vi "main.vi"() -> ()   [LabVIEW 2018]
uses:
  global.vi
  <vilib>/Instr/_visa.llb/VISA Configure Serial Port (Instr).vi
panel:
  out "当前位置":dbl
  out "频率test":string
  out "开关test":string
  out "步进电机test":string
  in  "停止":bool
  in  "改变开关":dbl=1.0 min=1.0 max=31.0 step=1.0
  in  "连接开关控制器":refnum<visa-resource-name>
  in  "连接步进电机控制器":refnum<visa-resource-name>
  in  "改变频率":dbl=24.0
  in  "改变位置":dbl
  in  "暂停":bool
  in  "开始":bool
  out "当前开关":dbl
  out "当前频率":dbl
  in  "扫描模式":string(combo)="多频多角度扫描"
  in  "测量距离/mm":dbl=150.0
  in  "频率步进/GHz":dbl=0.1
  in  "截止频率/GHz":dbl=30.0
  in  "起始频率/GHz":dbl=24.0
  in  "电机步进/mm":dbl=5.0
  in  "电机长度/mm":dbl=200.0
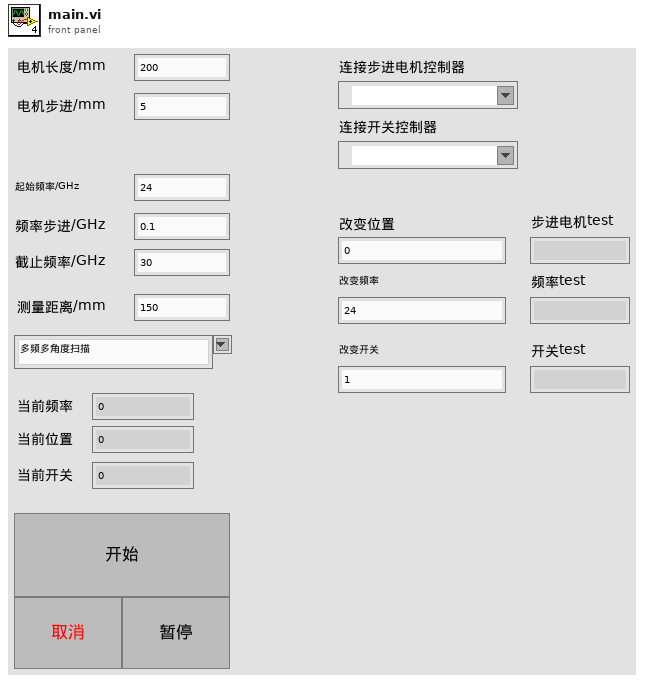
[diagram p1: front panel]
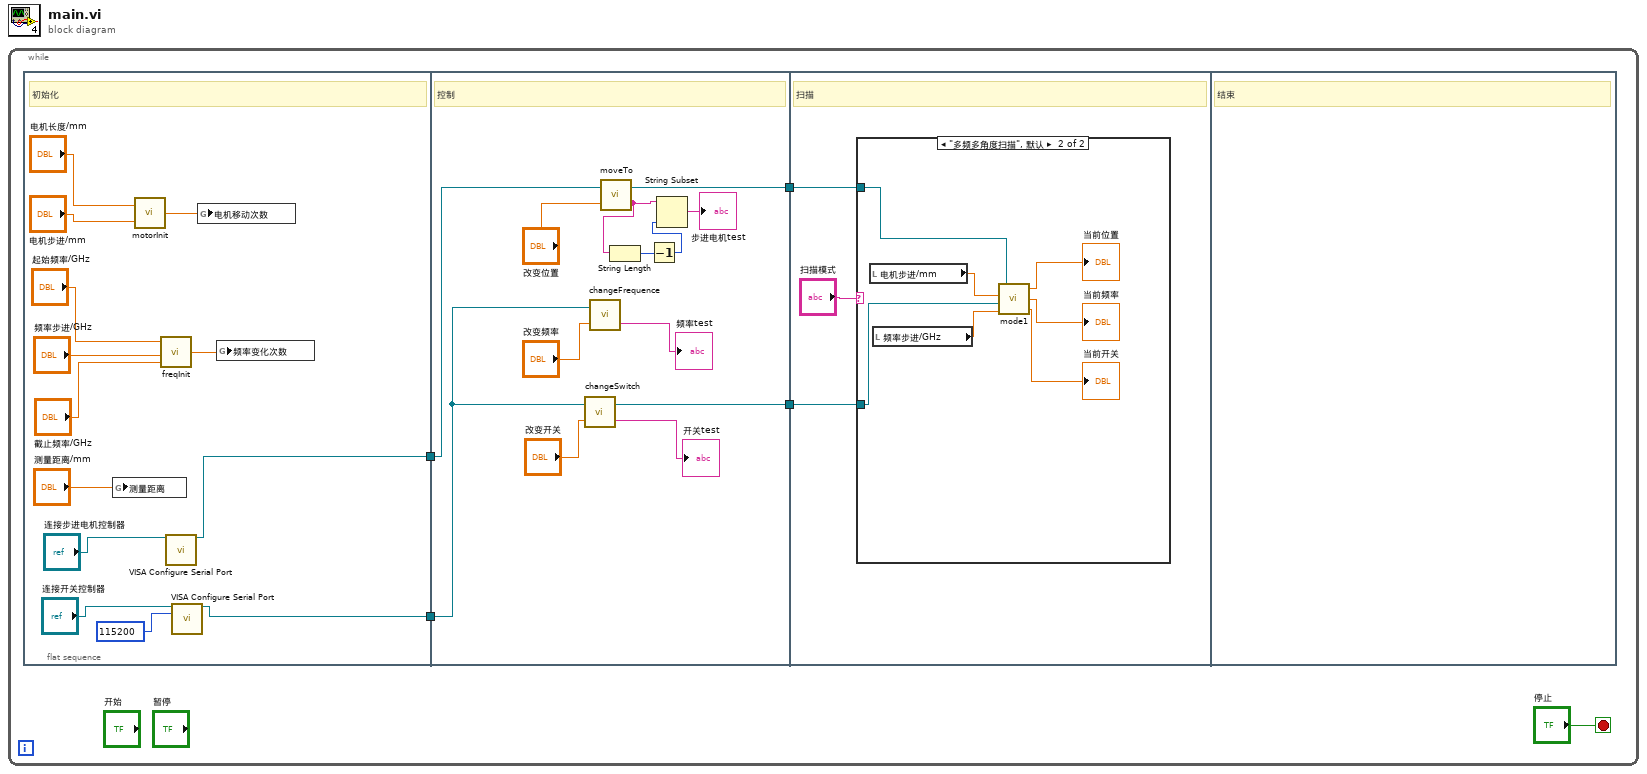
[diagram p0: block diagram]
diagram:
  n1 = while {
    stop <- "停止" stop-if-true
    n2 = flat-sequence {
      tunnel: [w6] -> w5
      tunnel: [w7] -> w4
      tunnel: w5 -> [w21]
      tunnel: w4 -> [w30]
      tunnel: [w20] -> w2
      tunnel: [w19] -> w1
      tunnel: w2 -> [w33]
      tunnel: w1 -> [w32]
      frame #0 {
        # "初始化"
        n3 = global write "global.vi" "测量距离"("测量距离/mm") -> ()
        n4 = call "motorInit.vi"("电机步进"="电机步进/mm", "电机长度"="电机长度/mm") -> ("电机移动次数"=w13:dbl)
        n5 = call "freqInit.vi"("频率终止"="截止频率/GHz", "频率步进"="频率步进/GHz", "频率起始"="起始频率/GHz") -> ("频率变化次数"=w17:dbl)
        n6 = call-poly "VISA Configure Serial Port"("VISA resource name"="连接步进电机控制器") -> ("VISA resource name out"=w6:refnum<visa-resource-name>)  [unwired: 13 in, 1 out]
        n7 = call-poly "VISA Configure Serial Port"("VISA resource name"="连接开关控制器", "baud rate (9600)"=115200) -> ("VISA resource name out"=w7:refnum<visa-resource-name>)  [unwired: 12 in, 1 out]
        n8 = global write "global.vi" "电机移动次数"(w13) -> ()
        n9 = global write "global.vi" "频率变化次数"(w17) -> ()
      }
      frame #1 {
        # "控制"
        n10 = call "changeSwitch.vi"("数值"="改变开关", "单片机串口"=w30) -> ("返回值"=→"开关test":string, "单片机串口 2"=w19:refnum<visa-resource-name>)
        n11 = call "changeFrequence.vi"("频率值"="改变频率", "单片机串口"=w30) -> ("字符串"=→"频率test":string)  [unwired: 1 out]
        n12 = call "moveTo.vi"("移动到位置"="改变位置", "步进电机控制器串口"=w21) -> ("字符串"=w24:string, "VISA资源名称"=w20:refnum<visa-resource-name>)
        n13 = String Length(string=w24) -> (length=w23:i32)
        n14 = Decrement(x=w23) -> (x-1=w22:i32)
        n15 = String Subset(string=w24, length (rest)=w22) -> (substring=→"步进电机test":string)  [unwired: 1 in]
      }
      frame #2 {
        # "扫描"
        n16 = case shown="\"多频多角度扫描\", 默认" "扫描模式" {
          tunnel: w33 -> [_ w41]
          tunnel: w32 -> [_ w40]
          frame "多频单角度扫描" {
          }
          frame "多频多角度扫描", Default {
            n17 = local read "电机步进/mm"() -> (w39:dbl)
            n18 = local read "频率步进/GHz"() -> (w38:dbl)
            n19 = call "mode1.vi"("步进频率"=w38, "单片机串口"=w40, "步进距离"=w39, "步进电机串口"=w41) -> ("当前开关"=→"当前开关":dbl, "当前频率"=→"当前频率":dbl, "当前位置"=→"当前位置":dbl)
          }
        }
      }
      frame #3 {
        # "结束"
      }
    }
  }
